vi "oopAPI_TX (UDP Port-Oriented)_MultiVL.vi"() -> ()   [LabVIEW 2020]
uses:
  src/_controls/comm_computedMAC-IP.ctl
  src/_controls/comm_udp_tx.ctl
  src/_controls/comm_config_vl_tx.ctl
  src/_polimorphicInstances/session/CreateSession(Tx-UDP Port-Oriented).vi
  src/bsp/AFDX_Transmit/Create Tx VL.vi
  src/_polimorphicInstances/udpPort/CreateUdpPort(TX-CommPort).vi
  src/AIM664LV.lvlib
panel:
  out "Duplicated":bool
  in  "VL Config":T1[](array[typedef]) {"NetSelect" items=["FDX_TX_FRAME_DLY_A"=0, "FDX_TX_FRAME_DLY_B"=1, "FDX_TX_FRAME_BOTH "=3, "FDX_TX_FRAME_ONLY_A"=4, "FDX_TX_FRAME_ONLY_B "=5]; "interfaceID" format="%.0b"}
  in  "CommPort Config":T2={"PortType"=enum."FDX_UDP_SAMPLING", "partitionID"=0, "SubVlId"=1, "UdpSrcPort"=0, "UdpDstPort"=0, "SampleRateMs"=128.0, "UdpNumBufMessages"=0, "UdpMaxMessageSize"=0}
  in  "millisecond multiple":u32=128
  in  "PortMap":u32
  out "size(s)":i32
  out "IndexCycleCount":u32[](array[numeric])
  out "MsgCount":u32[](array[numeric])
  out "CurrentIndex":u32[](array[numeric])
  out "BytesWritten":u32[](array[numeric])
  in  "port":u32
  in  "board":u32
  out "current time":timestamp=timestamp(3677762637.591913 s since 1904-01-01)
  out "current irig time":T3={"SignOut"=40, "DayOut"=1, "HourOut"=1, "MinOut"=28, "SecondOut"=39, "MilliSecOut"=539, "MicroSecOut"=300, "NanoSecOut"=0, "InfoOut"=0, "Mode"=3}
  out "CommPort Addresses":T4[](array[typedef]) {"MACsrc" format="%.0x"}
  in  "Data":u8[](array[numeric])=[255, 255, 255, 255, 255, 255, 255, 255, 255, 255, 255, 255, 255, 255, 255, 255, 255, 255, 255, 255, 255, 255, 255, 255, 255, 255, 255, 255, 255, 255, 255, 255, 255, 255, 255, 255, 255, 255, 255, 255, 255, 255, 255, 255, 255, 255, 255, 255, 255, 255, 255, 255, 255, 255, 255, 255, 255, 255, 255, 255, 255, 255, 255, 255, 255, 255, 255, 255, 255, 255, 255, 255, 255, 255, 255, 255, 255, 255, 255, 255, 255, 255, 255, 255, 255, 255, 255, 255, 255, 255, 255, 255, 255, 255, 255, 255, 255, 255, 255, 170] format="%.0x"
  in  "stop":bool
  out "PortInitOut":T5={"PortConfig"=0, "PortUsed"=1, "GlobalMemFree"=0, "SharedMemFree"=0} {"PortConfig" items=["FDX_SINGLE", "FDX_REDUNDANT"]}
  out "error out":errorcluster
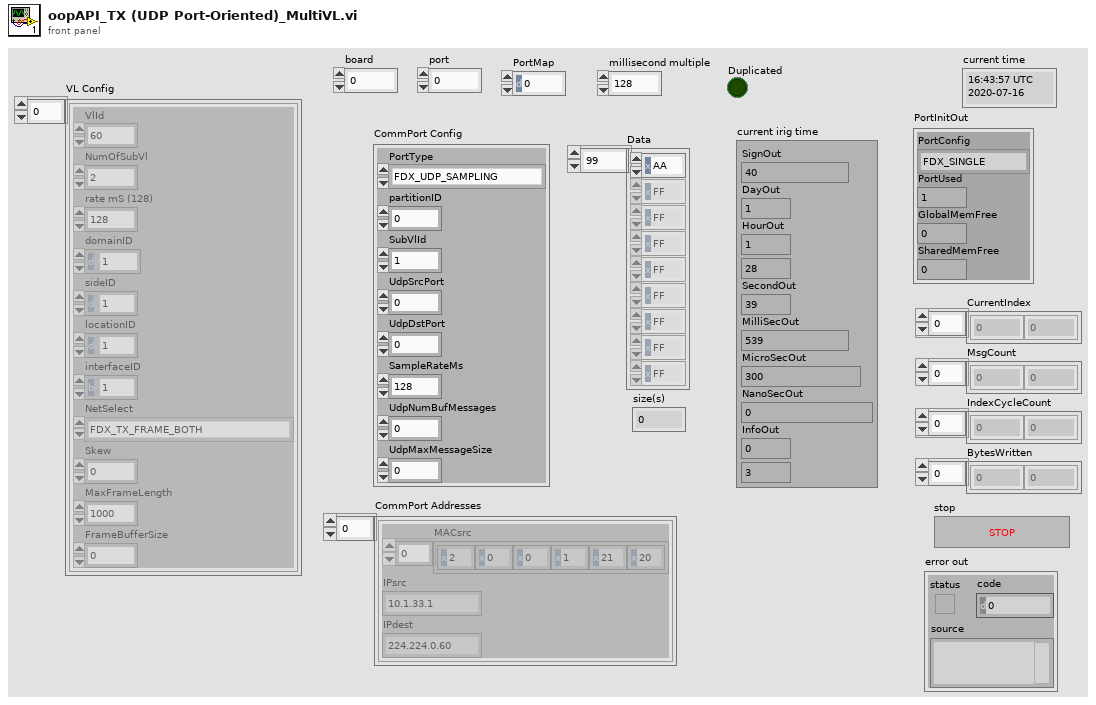
[diagram p1: front panel]
types:
  T1 = typedef "AIM664LV.lvlib/comm_config_vl_tx.ctl" = cluster{"VlId":u16, "NumOfSubVl":u16, "rate mS (128)":dbl, "domainID":u8, "sideID":u8, "locationID":u8, "interfaceID":u8, "NetSelect":u32, "Skew":u32, "MaxFrameLength":u32, "FrameBufferSize":u32}
  T2 = typedef "AIM664LV.lvlib/comm_udp_tx.ctl" = cluster{"PortType":enum16{"FDX_UDP_SAMPLING", "FDX_UDP_QUEUING"}, "partitionID":u8, "SubVlId":u8, "UdpSrcPort":u16, "UdpDstPort":u16, "SampleRateMs":dbl, "UdpNumBufMessages":u32, "UdpMaxMessageSize":u32}
  T3 = cluster{"SignOut":i32, "DayOut":u32, "HourOut":u32, "MinOut":u32, "SecondOut":u32, "MilliSecOut":u32, "MicroSecOut":u32, "NanoSecOut":u32, "InfoOut":u32, "Mode":u32}
  T4 = typedef "AIM664LV.lvlib/comm_computedMAC-IP.ctl" = cluster{"MACsrc":u8[], "IPsrc":string, "IPdest":string}
  T5 = cluster{"PortConfig":u32, "PortUsed":u32, "GlobalMemFree":u32, "SharedMemFree":u32}
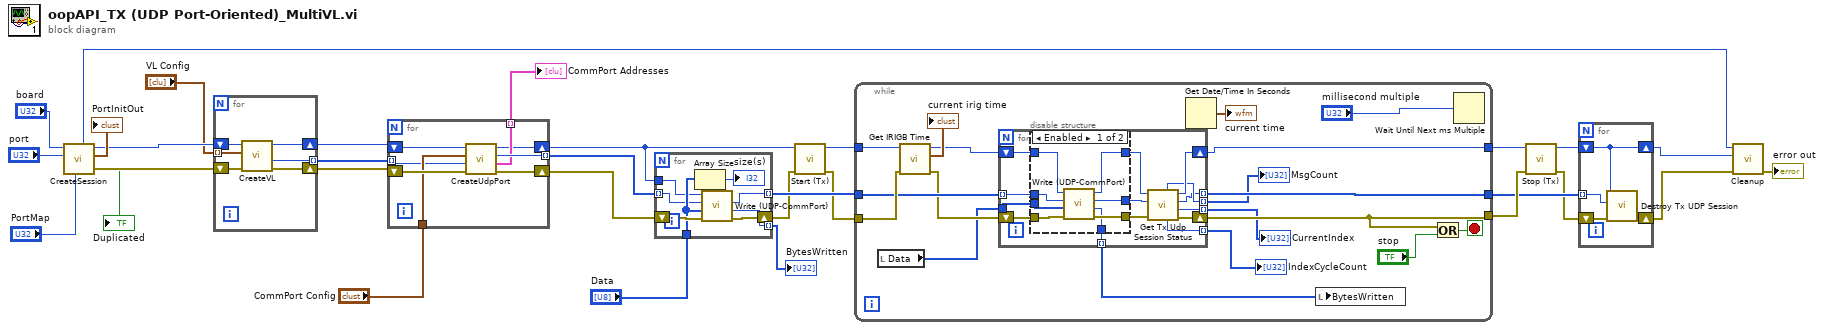
[diagram p0: block diagram]
diagram:
  n1 = call-poly "CreateSession.vi"("PortMap"="PortMap", "port"="port", "board"="board") -> ("error out"=w12:errorcluster, "PortInitOut"=→"PortInitOut":T5, "port handle out"=w13:u32, "Duplicated"=→"Duplicated":bool, "InstrumentHandle_board out"=w1:u32)  [unwired: 4 in]
  n2 = for {
    tunnel: [w33] -> w9 mode=indexing
    tunnel: "VL Config" -> [w32] mode=indexing
    shift-right: [w35] -> w11
    shift-left: w13 -> [w37]
    shift-right: [w34] -> w10
    shift-left: w12 -> [w36]
    n3 = call-poly "CreateVL.vi"("error in (no error)"=w36, "VL Config"=w32, "InstrumentHandle in"=w37) -> ("error out"=w34:errorcluster, "VlId"=w33:u16, "InstrumentHandle out"=w35:u32)  [unwired: 6 in]
  }
  n4 = for {
    tunnel: [w44] -> w29 mode=indexing
    tunnel: [w41] -> w25 mode=indexing
    shift-right: [w40] -> w5
    shift-left: w11 -> [w45]
    shift-right: [w43] -> w27
    shift-left: w10 -> [w42]
    tunnel: w9 -> [w38] mode=indexing
    tunnel: "CommPort Config" -> [w39]
    n5 = call-poly "CreateUdpPort.vi"("error in (no error)"=w42, "VlId"=w38, "CommPort Config"=w39, "port handle in"=w45) -> ("error out"=w43:errorcluster, "computedAddresses"=w41:T4, "commPort handle out"=w44:u32, "port handle out"=w40:u32)  [unwired: 4 in]
  }
  "CommPort Addresses" <- w25
  n6 = for {
    tunnel: "Data" -> [w49]
    tunnel: [w51] -> w15 mode=indexing
    shift-right: [w52] -> w23
    shift-left: w27 -> [w53]
    tunnel: w29 -> [w48] mode=indexing
    tunnel: [w46] -> w28 mode=indexing
    tunnel: w5 -> [w47]
    n7 = Array Size(array=w49) -> (size(s)=→"size(s)":i32)
    n8 = call "Write (UDP-CommPort).vi"("error in (no error)"=w53, "Data"=w49, "UdpHandle in"=w48, "InstrumentHandle_port in"=w47) -> ("error out"=w52:errorcluster, "BytesWritten"=w51:u32, "UdpHandle out"=w46:u32)  [unwired: 4 in, 1 out]
  }
  "BytesWritten" <- w15
  n9 = call "Start (Tx).vi"("error in (no error)"=w23, "InstrumentHandle_port in"=w5) -> ("error out"=w22:errorcluster, "InstrumentHandle_port out"=w21:u32)  [unwired: 8 in]
  n10 = while {
    tunnel: w22 -> [w67]
    tunnel: w28 -> [w59]
    tunnel: w21 -> [w68]
    tunnel: [w54] -> w24
    tunnel: [w64] -> w18
    tunnel: [w63] -> w19
    stop <- w70 stop-if-true
    n11 = local read "Data"() -> (w56:u8[])
    n12 = call "Get IRIGB Time.vi"("error in (no error)"=w67, "InstrumentHandle_board in"=w68) -> ("error out"=w58:errorcluster, "Curent Irig Time"=→"current irig time":T3, "InstrumentHandle_board out"=w55:u32)  [unwired: 7 in]
    n13 = for {
      tunnel: [w74] -> w64 mode=indexing
      tunnel: [w73] -> w62 mode=indexing
      tunnel: [w75] -> w61 mode=indexing
      tunnel: [w72] -> w60 mode=indexing
      tunnel: w59 -> [w84] mode=indexing
      tunnel: [w79] -> w57 mode=indexing
      tunnel: w56 -> [w81]
      shift-right: [w85] -> w63
      shift-left: w58 -> [w83]
      shift-right: [w76] -> w54
      shift-left: w55 -> [w80]
      n14 = disable-structure shown="Enabled" {
        disable-tunnel: w84 -> [w90 w95]
        disable-tunnel: w83 -> [w93 w94]
        disable-tunnel: [w92 w94] -> w82
        disable-tunnel: [w86 w95] -> w78
        disable-tunnel: w81 -> [w91 _]
        disable-tunnel: w80 -> [w89 _]
        disable-tunnel: [w88 _] -> w79
        disable-tunnel: [w87 _] -> w77
        frame Enabled {
          n15 = call "Write (UDP-CommPort).vi"("error in (no error)"=w93, "Data"=w91, "UdpHandle in"=w90, "InstrumentHandle_port in"=w89) -> ("error out"=w92:errorcluster, "BytesWritten"=w88:u32, "UdpHandle out"=w86:u32, "InstrumentHandle_port out"=w87:u32)  [unwired: 4 in]
        }
        frame Disabled {
        }
      }
      n16 = call "Get Tx Udp Session Status.vi"("error in (no error)"=w82, "UdpHandle in"=w78, "InstrumentHandle_port in"=w77) -> ("error out"=w85:errorcluster, "CurrentIndex"=w73:u32, "UdpHandle out"=w74:u32, "InstrumentHandle_port out"=w76:u32, "IndexCycleCount"=w72:u32, "MsgCount"=w75:u32)  [unwired: 3 in]
    }
    "CurrentIndex" <- w62
    "MsgCount" <- w61
    "IndexCycleCount" <- w60
    n17 = Get Date/Time In Seconds() -> (seconds since 1Jan1904=→"current time":timestamp)
    n18 = local write "BytesWritten"(w57) -> ()
    n19 = Or(x=w63, y="stop") -> (x .or. y?=w70:bool)
    n20 = Wait Until Next ms Multiple(millisecond multiple="millisecond multiple") -> ()  [unwired: 1 out]
  }
  n21 = call "Stop (Tx).vi"("error in (no error)"=w19, "InstrumentHandle_port in"=w24) -> ("error out"=w17:errorcluster, "InstrumentHandle_port out"=w4:u32)  [unwired: 8 in]
  n22 = for {
    tunnel: w18 -> [w97] mode=indexing
    shift-right: [w98] -> w16
    shift-left: w17 -> [w99]
    shift-right: [w96] -> w3
    shift-left: w4 -> [w96]
    n23 = call "Destroy Tx UDP Session.vi"("error in (no error)"=w99, "UdpHandle in"=w97, "InstrumentHandle_port in"=w96) -> ("error out"=w98:errorcluster)  [unwired: 7 in, 1 out]
  }
  n24 = call "Cleanup.vi"("error in (no error)"=w16, "InstrumentHandle_port in"=w3, "InstrumentHandle_board in"=w1) -> ("error out"=→"error out":errorcluster)  [unwired: 8 in]
